vi "DATA BASE.vi"() -> ()   [LabVIEW 2017]
panel:
  out "deleted portion":T1(array[cluster])
  out "array w/ subset deleted":T1(array[cluster])
  out "output array":T1(array[cluster])
  in  "new element/subarray":T2
  in  "Array":T1(array[cluster])
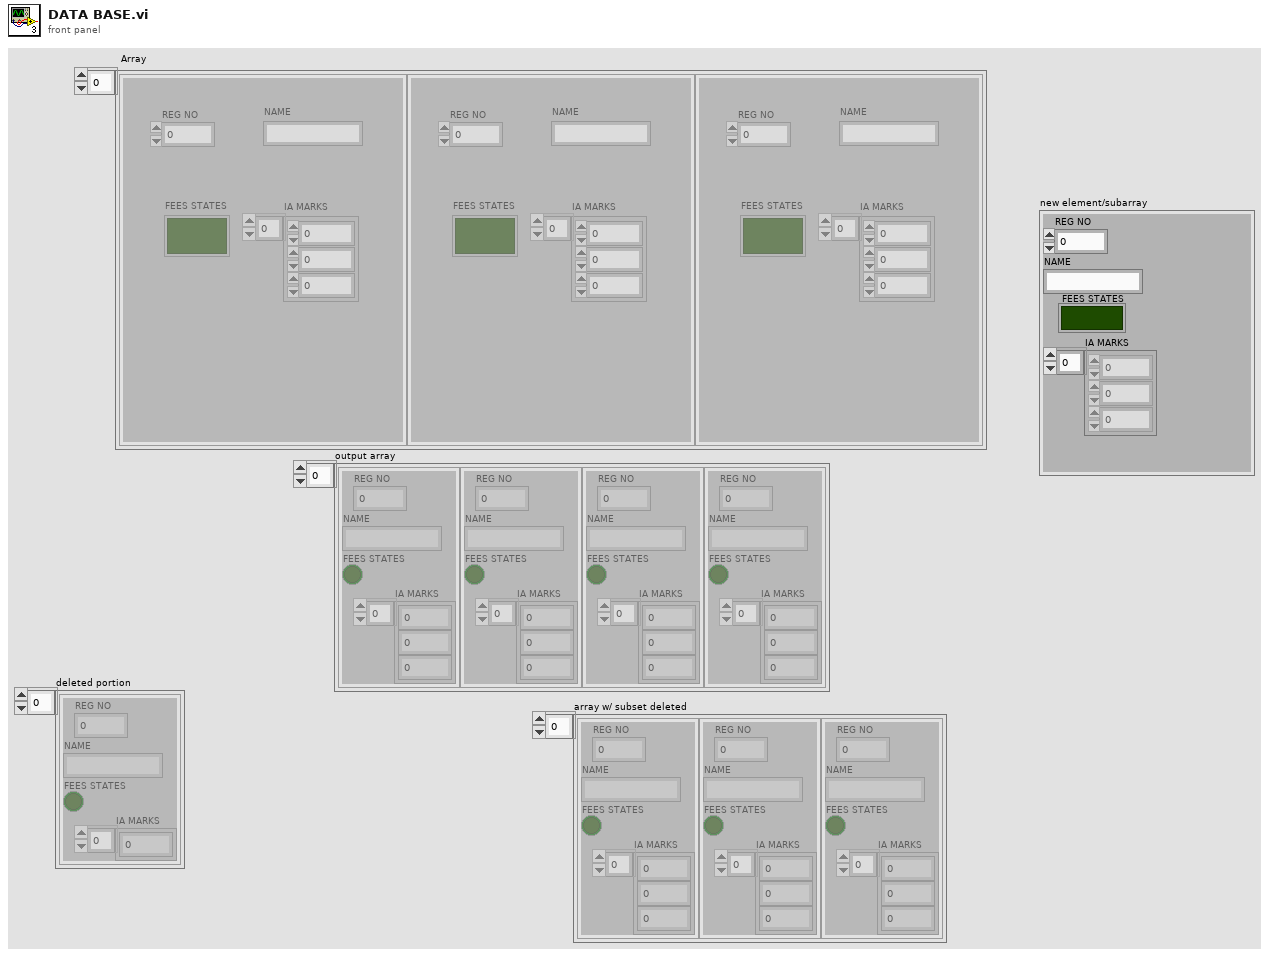
[diagram p1: front panel]
types:
  T1 = cluster{"REG NO":dbl, "NAME":string, "FEES STATES":bool, "IA MARKS":dbl[]}[]
  T2 = cluster{"REG NO":dbl, "NAME":string, "FEES STATES":bool, "IA MARKS":dbl[]}
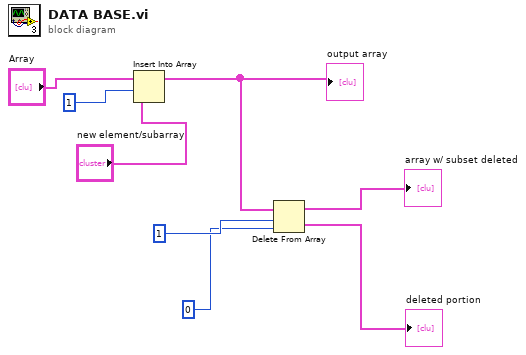
[diagram p0: block diagram]
diagram:
  n1 = Insert Into Array "Insert Into Array"(array="Array", index=1, new element="new element/subarray") -> (w5:T1)
  "output array" <- w5
  n2 = Delete From Array(array=w5, length=1, index=0) -> (deleted portion=→"deleted portion":T1, array with subset deleted=→"array w/ subset deleted":T1)
